vi "Get Properties by Class Hierarchy_2.vi"(8 "error in (no error)":errorcluster, 11 "Class ID":string) -> (0 "error out":errorcluster, 2 "Classes Processed":string[](array[string]), 3 "Properties by Class Hierarchy":T1(array[cluster]))   [LabVIEW 2023]
doc: "<b> </b> <b> </b>\n© 2017 Q Software Innovations, LLC\nwritten by Quentin \"Q\" Alldredge\nproduced in LabVIEW 2015\n\nsupport@qsoftwareinnovations.com\nwww.qsoftwareinnovations.com\n\nAll rights reserved.\n\nRedistribution and use in source and binary forms, with or without modification, are permitted provided that the following conditions are met:\n\n * Redistributions of source code must retain the above copyright notice, this list of conditions and the following disclaimer.\n * Redistributions in binary form must reproduce the above copyright notice, this list of conditions and the following disclaimer in the documentation and/or other materials provided with the distribution.\n * Neither the name of Q Software Innovations, LLC. nor the names of its contributors may be used to endorse or promote products derived from this software without specific prior written permission.\n\nTHIS SOFTWARE IS PROVIDED BY THE COPYRIGHT HOLDERS AND CONTRIBUTORS \"AS IS\" AND ANY EXPRESS OR IMPLIED WARRANTIES, INCLUDING, BUT NOT LIMITED TO, THE IMPLIED WARRANTIES OF MERCHANTABILITY AND FITNESS FOR A PARTICULAR PURPOSE ARE DISCLAIMED. IN NO EVENT SHALL THE COPYRIGHT OWNER OR CONTRIBUTORS BE LIABLE FOR ANY DIRECT, INDIRECT, INCIDENTAL, SPECIAL, EXEMPLARY, OR CONSEQUENTIAL DAMAGES (INCLUDING, BUT NOT LIMITED TO, PROCUREMENT OF SUBSTITUTE GOODS OR SERVICES; LOSS OF USE, DATA, OR PROFITS; OR BUSINESS INTERRUPTION) HOWEVER CAUSED AND ON ANY THEORY OF LIABILITY, WHETHER IN CONTRACT, STRICT LIABILITY, OR TORT (INCLUDING NEGLIGENCE OR OTHERWISE) ARISING IN ANY WAY OUT OF THE USE OF THIS SOFTWARE, EVEN IF ADVISED OF THE POSSIBILITY OF SUCH DAMAGE."
panel:
  out "exe time (ms)":u32
  out "size(s)":i32
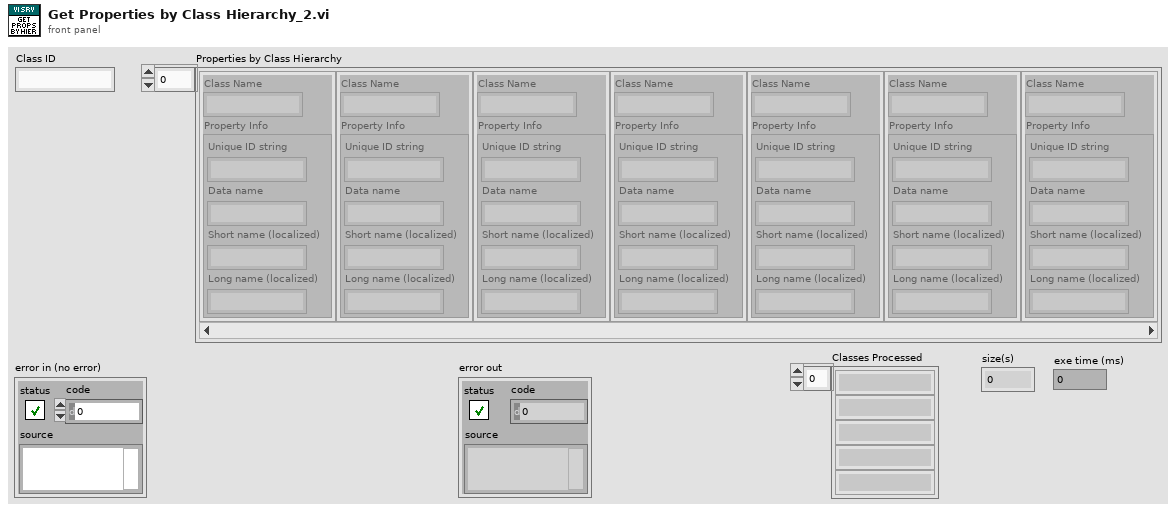
[diagram p1: front panel]
types:
  T1 = cluster{"Class Name":string, "Property Info":cluster{"Unique ID string":string, "Data name":string, "Short name (localized)":string, "Long name (localized)":string}}[]
  T2 = cluster{"Unique ID string":string, "Data name":string, "Short name (localized)":string, "Long name (localized)":string}[]
  T3 = cluster{"Unique ID string":string, "Parent ID string":string, "Class Name (unlocalized)":string, "Class Name (localized)":string}
  T4 = cluster{"Class Name (unlocalized)":string, "Property/Method Info":cluster{"Unique ID string":string, "Data name":string, "Short name (localized)":string, "Long name (localized)":string}}
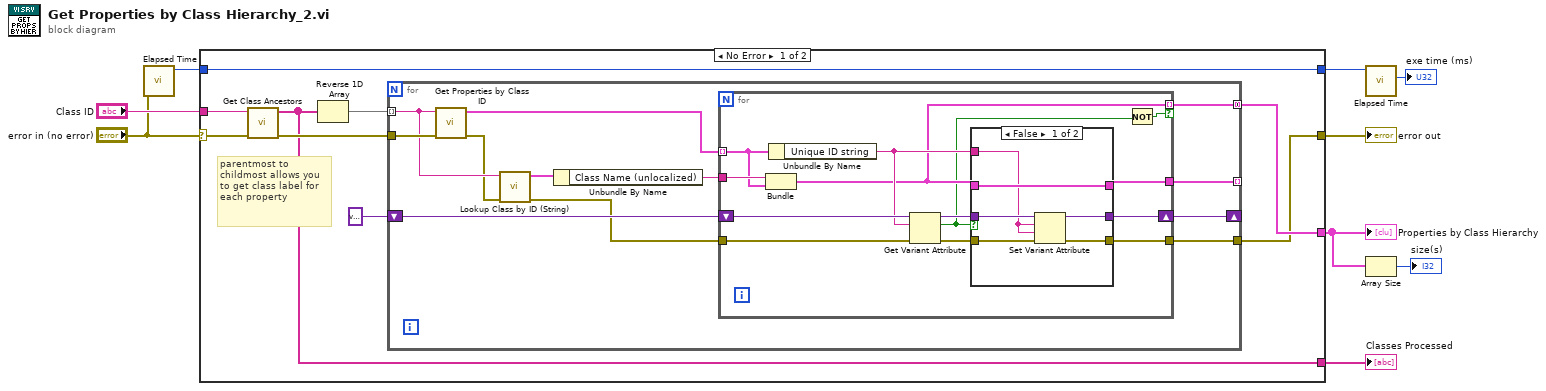
[diagram p0: block diagram]
diagram:
  n1 = call "Elapsed Time.vi"("error in"="error in (no error)") -> ("millisecond timer value"=w5:u32)  [unwired: 6 in, 4 out]
  n2 = case shown="No Error" "error in (no error)" {
    selector: "error in (no error)" -> [w18 w54]
    tunnel: [w10 w54] -> w9
    tunnel: "Class ID" -> [w17 _]
    tunnel: [w11 _] -> w2
    tunnel: w5 -> [w14 w53]
    tunnel: [w14 w53] -> w4
    tunnel: [w12 _] -> w1
    frame No Error {
      # "parentmost to childmost allows you to get class label for each property"
      n3 = call "Get Class Ancestors.vi"("error in (no error)"=w18, "Class ID"=w17) -> ("error out"=w16:errorcluster, "Class Ancestor IDs[]"=w12:string[])  [unwired: 8 in]
      n4 = Reverse 1D Array(array=w12) -> (reversed array=w13:string[])
      n5 = for {
        tunnel: w16 -> [w30]
        tunnel: w13 -> [w26] mode=indexing
        shift-right: [w28] -> _
        shift-left: variant -> [w29]
        tunnel: [w21] -> _ mode=indexing
        tunnel: [w20] -> w10
        tunnel: [w19] -> w11 mode=concatenating
        n6 = call "Get Properties by Class ID.vi"("error in (no error)"=w30, "Class ID"=w26) -> ("error out"=w25:errorcluster, "Properties[]"=w27:T2)  [unwired: 8 in]
        n7 = call "Lookup Class by ID (String).vi"("error in (no error)"=w25, "Class ID"=w26) -> ("error out"=w24:errorcluster, "Class Information"=w23:T3)  [unwired: 7 in, 1 out]
        n8 = Unbundle By Name(w23) -> ("Class Name (unlocalized)"=w22:string)
        n9 = for {
          shift-right: [w41] -> w28
          shift-left: w29 -> [w43]
          tunnel: w27 -> [w36] mode=indexing
          tunnel: w24 -> [w42]
          tunnel: w22 -> [w37]
          tunnel: [w35] -> w21
          tunnel: [w34] -> w20
          tunnel: [w33] -> w19 mode=indexing if=w31
          n10 = Bundle("Class Name (unlocalized)"=w37, "Property/Method Info"=w36) -> (w33:T4)  [unwired: 1 in]
          n11 = Unbundle By Name(w36) -> ("Unique ID string"=w39:string)
          n12 = Get Variant Attribute(Variant=w43, name=w39, error in=w42) -> (duplicate Variant=w40:variant, found=w32:bool, error out=w38:errorcluster)  [unwired: 1 in, 1 out]
          n13 = case shown="False" w32 {
            tunnel: [w48 w52] -> w41
            tunnel: w40 -> [w49 w52]
            tunnel: w39 -> [w44 _]
            tunnel: w38 -> [w47 w50]
            tunnel: w33 -> [w46 w51]
            tunnel: [w46 w51] -> w35
            tunnel: [w45 w50] -> w34
            frame False {
              n14 = Set Variant Attribute(Variant=w49, name=w44, value=w44, error in=w47) -> (Variant out=w48:variant, error out=w45:errorcluster)  [unwired: 1 out]
            }
            frame True {
            }
          }
          n15 = Not(x=w32) -> (.not. x?=w31:bool)
        }
      }
    }
    frame Error {
    }
  }
  "error out" <- w9
  "Properties by Class Hierarchy" <- w2
  "Classes Processed" <- w1
  n16 = call "Elapsed Time.vi"("past time"=w4) -> ("elapsed time (ms)"=→"exe time (ms)":u32)  [unwired: 6 in, 4 out]
  n17 = Array Size(array=w2) -> (size(s)=→"size(s)":i32)
